vi "DeviceValveDiagnostics.vi"(1 "Sensor Values":dbl[](array[numeric])) -> (0 "?":bool, 2 "Power Connected":bool, 3 "?":bool, 4 "?":bool, 5 "?":bool, 6 "?":bool, 7 "?":bool, 8 "?":bool, 9 "?":bool)   [LabVIEW 2021]
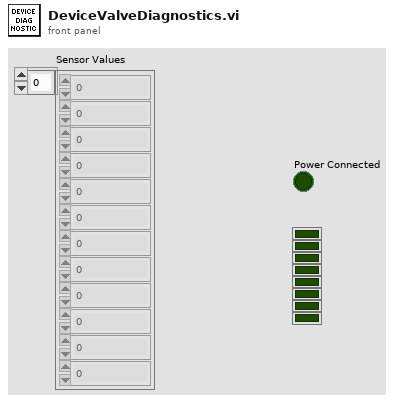
[diagram p1: front panel]
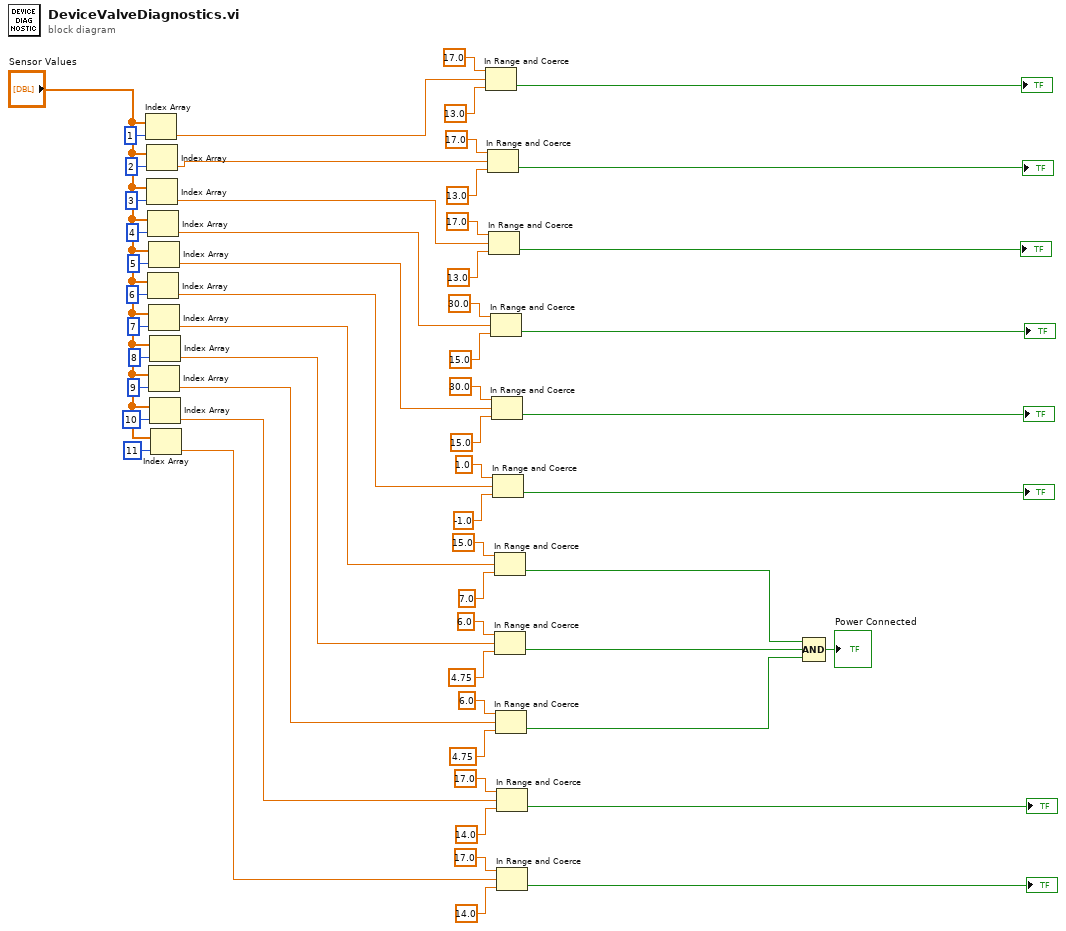
[diagram p0: block diagram]
diagram:
  n1 = Index Array(array="Sensor Values", index=1) -> (element=w45:dbl)
  n2 = Index Array(array="Sensor Values", index=2) -> (element=w38:dbl)
  n3 = Index Array(array="Sensor Values", index=3) -> (element=w37:dbl)
  n4 = Index Array(array="Sensor Values", index=4) -> (element=w34:dbl)
  n5 = Index Array(array="Sensor Values", index=6) -> (element=w22:dbl)
  n6 = Index Array(array="Sensor Values", index=5) -> (element=w31:dbl)
  n7 = Index Array(array="Sensor Values", index=7) -> (element=w7:dbl)
  n8 = Index Array(array="Sensor Values", index=9) -> (element=w5:dbl)
  n9 = Index Array(array="Sensor Values", index=8) -> (element=w6:dbl)
  n10 = Index Array(array="Sensor Values", index=10) -> (element=w14:dbl)
  n11 = Index Array(array="Sensor Values", index=11) -> (element=w15:dbl)
  n12 = In Range and Coerce(upper limit=17.0, x=w45, lower limit=13.0) -> (In Range?=→"?":bool)  [unwired: 1 out]
  n13 = In Range and Coerce(upper limit=17.0, x=w38, lower limit=13.0) -> (In Range?=→"?":bool)  [unwired: 1 out]
  n14 = In Range and Coerce(upper limit=17.0, x=w37, lower limit=13.0) -> (In Range?=→"?":bool)  [unwired: 1 out]
  n15 = In Range and Coerce(upper limit=30.0, x=w34, lower limit=15.0) -> (In Range?=→"?":bool)  [unwired: 1 out]
  n16 = In Range and Coerce(upper limit=30.0, x=w31, lower limit=15.0) -> (In Range?=→"?":bool)  [unwired: 1 out]
  n17 = In Range and Coerce(upper limit=1.0, x=w22, lower limit=-1.0) -> (In Range?=→"?":bool)  [unwired: 1 out]
  n18 = In Range and Coerce(upper limit=15.0, x=w7, lower limit=7.0) -> (In Range?=w4:bool)  [unwired: 1 out]
  n19 = In Range and Coerce(upper limit=6.0, x=w6, lower limit=4.75) -> (In Range?=w3:bool)  [unwired: 1 out]
  n20 = In Range and Coerce(upper limit=6.0, x=w5, lower limit=4.75) -> (In Range?=w2:bool)  [unwired: 1 out]
  n21 = In Range and Coerce(upper limit=17.0, x=w14, lower limit=14.0) -> (In Range?=→"?":bool)  [unwired: 1 out]
  n22 = In Range and Coerce(upper limit=17.0, x=w15, lower limit=14.0) -> (In Range?=→"?":bool)  [unwired: 1 out]
  n23 = Compound Arithmetic op=AND(w4, w3, w2) -> (→"Power Connected":bool)
